vi "FindItem.vi"(7 "Item Name":string, 8 "error in (no error)":errorcluster, 10 "StructuredDataContainer":variant, 11 "BlueJSONTextSerializer in":refnum<class "BlueJSONTextSerializer.lvclass">) -> (0 "error out":errorcluster, 1 "Found":bool, 2 "StructuredDataItem":variant, 3 "BlueJSONTextSerializer out":refnum<class "BlueJSONTextSerializer.lvclass">)   [LabVIEW 2019, in "BlueJSONTextSerializer.lvlib" / "BlueJSONTextSerializer.lvclass"]
uses:
  BlueJSONTextSerializer.lvclass
  StructuredData.ctl
  <userlib>/Blue Origin/Blue JSONtext/String Subset.vi
  <userlib>/Blue Origin/Blue JSONtext/Parsing/Parse Full Path or Item Name.vi
  <userlib>/Blue Origin/Blue JSONtext/Next JSON Value.vi
  <userlib>/Blue Origin/Blue JSONtext/support/Error Cluster From Code.vi
  <userlib>/Blue Origin/Blue JSONtext/Offset/Find Item Locations by Path.vi
  <vilib>/JDP Science/JSONtext/JSONtext.lvlib
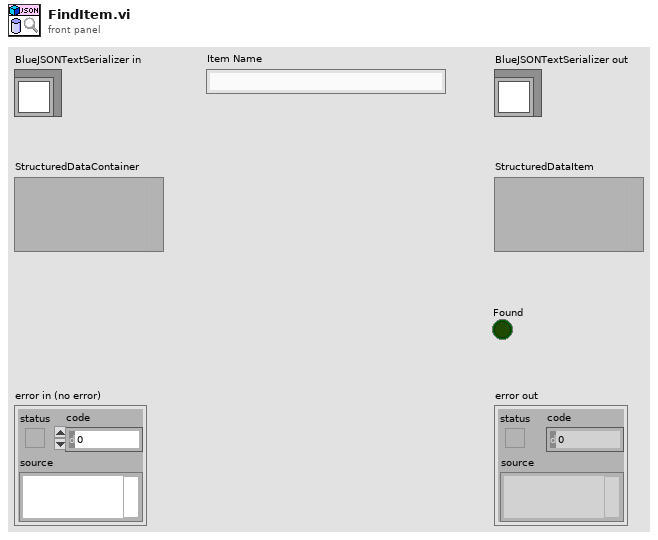
[diagram p1: front panel]
types:
  T1 = typedef "BlueJSONTextSerializer.lvlib/BlueJSONTextSerializer.lvclass/StructuredData.ctl" = cluster{"JSON":string, "Offset":i32}
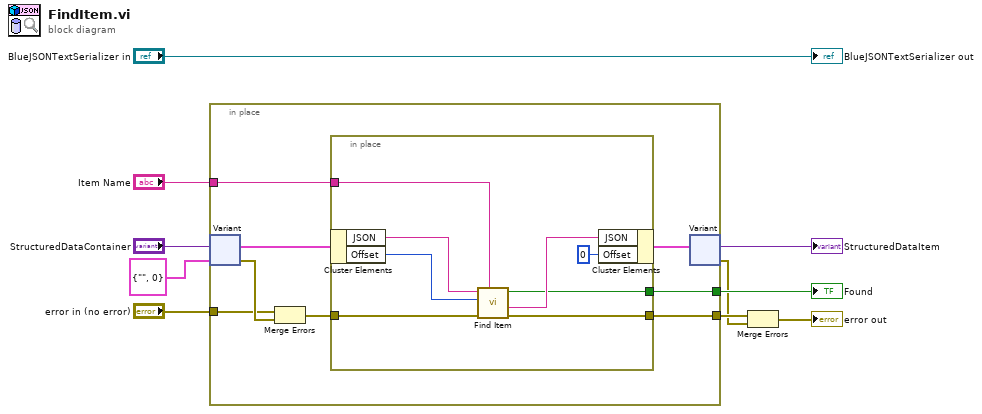
[diagram p0: block diagram]
diagram:
  n1 = in-place {
    in-place-border: "Item Name" -> [w18]
    in-place-border: [w17] -> w3
    in-place-border: [w16] -> w8
    in-place-border: "error in (no error)" -> [w12]
    n2 = in-place-variant #1("StructuredDataContainer", T1 {"JSON"="", "Offset"=0} ("Cluster")) -> (w15:T1, w14:errorcluster)
    n3 = Merge Errors(w12, w14) -> (w13:errorcluster)
    n4 = in-place {
      in-place-border: w18 -> [w23]
      in-place-border: w13 -> [w22]
      in-place-border: [w21] -> w17
      in-place-border: [w19] -> w16
      n5 = in-place-cluster #2(w15) -> ("JSON"=w25:string, "Offset"=w24:i32)
      n6 = call <vilib>:"Find Item.vi"("$Path or Item Name"=w23, "error in (no error)"=w22, "Offset"=w24, "JSON"=w25) -> ("error out"=w21:errorcluster, "<JSON>"=w20:string, "Found"=w19:bool)  [unwired: 4 in, 1 out]
      n7 = in-place-cluster #2("JSON"=w20, "Offset"=0) -> (w11:T1)
    }
    n8 = in-place-variant #1(w11) -> (→"StructuredDataItem":variant, w2:errorcluster)
  }
  "Found" <- w8
  n9 = Merge Errors(w3, w2) -> (→"error out":errorcluster)
  "BlueJSONTextSerializer out" <- "BlueJSONTextSerializer in"
